vi "Auto Path Names.vi"() -> (3 "Path Names":string[](array[string]))   [LabVIEW 2019]
uses:
  <vilib>/Rock Robotics/Network Tables/NT Read String.vi
  Framework/Robot Global Data.vi
  e9e0159d-0599-4be8-aab2-42ac49d9f226.vi
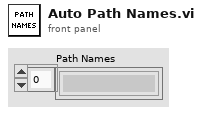
[diagram p1: front panel]
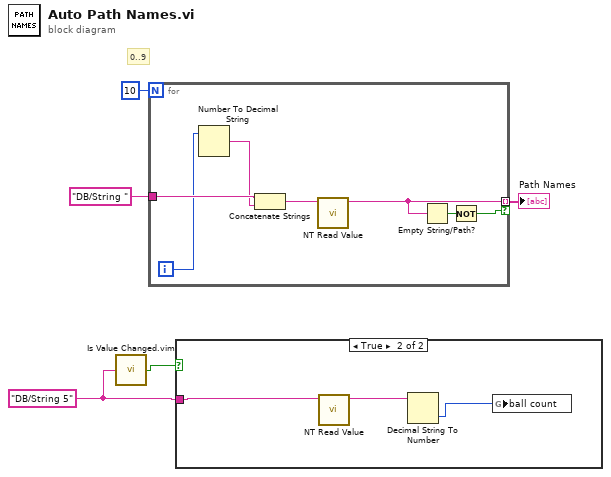
[diagram p0: block diagram]
diagram:
  w2 = "DB/String 5"
  # "0..9"
  n1 = call "Is Value Changed.vim"("value"=w2) -> ("changed or first call?"=w1:bool)
  n2 = for {
    N: 10 -> [_]
    tunnel: "DB/String " -> [w12]
    tunnel: [w9] -> w3 mode=indexing if=w7
    i -> [w6]
    n3 = Number To Decimal String(number=w6) -> (decimal integer string=w11:string)  [unwired: 1 in]
    n4 = Concatenate Strings(w12, w11) -> (w10:string)
    n5 = call-poly <vilib>:"NT Read Value.vi"("Name"=w10) -> ("String"=w9:string)  [unwired: 9 in, 1 out]
    n6 = Empty String/Path?(string/path=w9) -> (empty?=w8:bool)
    n7 = Not(x=w8) -> (.not. x?=w7:bool)
  }
  "Path Names" <- w3
  n8 = case shown="True" w1 {
    tunnel: w2 -> [_ w13]
    frame False {
    }
    frame True {
      n9 = call-poly <vilib>:"NT Read Value.vi"("Name"=w13) -> ("String"=w15:string)  [unwired: 9 in, 1 out]
      n10 = Decimal String To Number(string=w15) -> (number=w14:i32)  [unwired: 2 in, 1 out]
      n11 = global write "Robot Global Data.vi" "ball count"(w14) -> ()
    }
  }
